vi "Rotate_DBL.vi"(7 "Direction of Rotation":T1, 8 "error in (no error)":errorcluster, 10 "Angle (degrees)":dbl, 11 "CartesianVector in":refnum<class "CartesianVector.lvclass">) -> (0 "error out":errorcluster, 3 "CartesianVector out":refnum<class "CartesianVector.lvclass">)   [LabVIEW 2011, in "CartesianVector.lvclass"]
doc: "Takes in a CartesianVector object as well as an angle and a direction of rotation. Outputs a new CartesianVector object that has been rotated."
uses:
  CartesianVector.lvclass
  PolarVector/PolarVector.lvclass
  TypeDefs/DirectionOfRotation.ctl
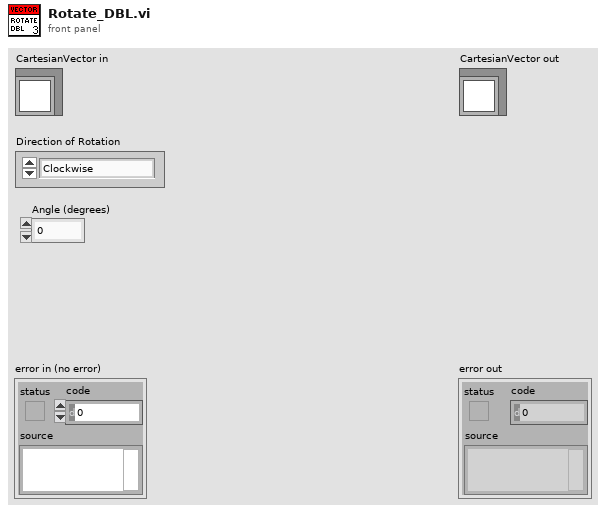
[diagram p1: front panel]
types:
  T1 = typedef "DirectionOfRotation.ctl" = enum16{"Clockwise", "Counter-Clockwise"}
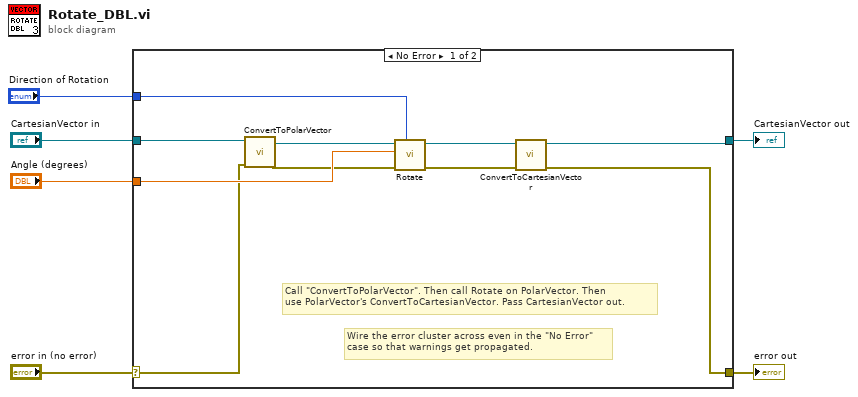
[diagram p0: block diagram]
diagram:
  n1 = case shown="No Error" "error in (no error)" {
    selector: "error in (no error)" -> [w7 w17]
    tunnel: [w9 w18] -> w4
    tunnel: "CartesianVector in" -> [w16 w18]
    tunnel: "Direction of Rotation" -> [w15 _]
    tunnel: "Angle (degrees)" -> [w13 _]
    tunnel: [w8 w17] -> w1
    frame No Error {
      # "Call \"ConvertToPolarVector\". Then call Rotate on PolarVector. Then\nuse PolarVector's ConvertToCartesianVector. Pass CartesianVector out."
      # "Wire the error cluster across even in the \"No Error\"\ncase so that warnings get propagated."
      n2 = call "ConvertToPolarVector.vi"("error in (no error)"=w7, "CartesianVector in"=w16) -> ("error out"=w12:errorcluster, "PolarVector.lvclass"=w14:refnum<class "PolarVector.lvclass">)  [unwired: 8 in]
      n3 = call-poly "Rotate.vi"("Direction of Rotation"=w15, "error in (no error)"=w12, "Angle (degrees)"=w13, "PolarVector in"=w14) -> ("error out"=w10:errorcluster, "PolarVector out"=w11:refnum<class "PolarVector.lvclass">)  [unwired: 6 in]
      n4 = call "ConvertToCartesianVector.vi"("error in (no error)"=w10, "PolarVector in"=w11) -> ("error out"=w8:errorcluster, "CartesianVector.lvclass"=w9:refnum<class "CartesianVector.lvclass">)  [unwired: 8 in]
    }
    frame Error {
    }
  }
  "error out" <- w1
  "CartesianVector out" <- w4
